vi "Convert Cartesian to Direct.vi"(8 "Lattice vector c":dbl[](array[numeric])=[0.0, 0.0, 22.8956], 9 "Lattice vector b":dbl[](array[numeric])=[0.0, 8.0948, 0.0], 10 "Lattice vector a":dbl[](array[numeric])=[4.67354, 0.0, 0.0], 11 "Positions (Cartesian)":dbl[][](array[numeric])) -> (3 "Positions (Direct)":dbl[][](array[numeric]))   [LabVIEW 2010]
uses:
  <vilib>/Analysis/baseanly.llb/Real Inverse Matrix.vi
  <vilib>/Analysis/baseanly.llb/A x Vector.vi
  <vilib>/Analysis/NI_AALBase.lvlib
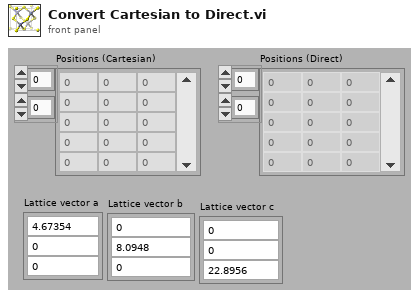
[diagram p1: front panel]
types:
  T1 = typedef "NI_Matrix.lvlib/RealMatrix.ctl" = dbl[][]
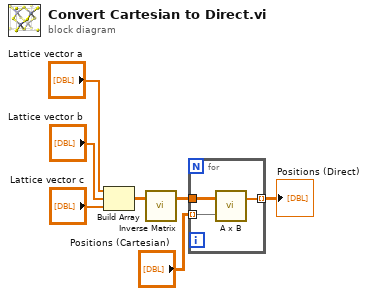
[diagram p0: block diagram]
diagram:
  n1 = Build Array("Lattice vector a", "Lattice vector b", "Lattice vector c") -> (w7:T1)
  n2 = call-poly <vilib>:"Inverse Matrix.vi"("Input Matrix"=w7) -> ("Inverse Matrix"=w3:T1)  [unwired: 1 in, 1 out]
  n3 = for {
    tunnel: w3 -> [w10]
    tunnel: "Positions (Cartesian)" -> [w9] mode=indexing
    tunnel: [w8] -> w1 mode=indexing
    n4 = call-poly <vilib>:"A x B.vi"("Vector"=w9, "A"=w10) -> ("A x Vector"=w8:dbl[])  [unwired: 1 out]
  }
  "Positions (Direct)" <- w1
